vi "Read Lump Data.vi"(8 "Lumps Directory IN":T1[](array[typedef]), 9 "start index (0)":i32, 10 "Lump Name":string, 11 "Input U8":u8[](array[numeric])) -> (0 "Lumps Directory OUT":T1[](array[typedef]), 1 "Lump DATA OUT":u8[](array[numeric]), 2 "Found?":bool, 3 "Output U8":u8[](array[numeric]))   [LabVIEW 2017]
uses:
  Lumps.ctl
panel:
  # "This will check the lump list for the lump name, get the offset and the length on the U8 data file and return the data of the lump"
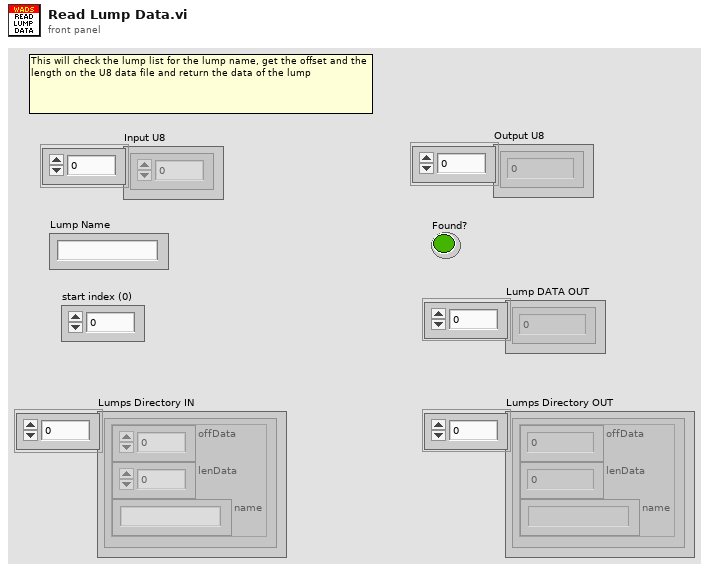
[diagram p1: front panel]
types:
  T1 = typedef "Lumps.ctl" = cluster{"offData":i32, "lenData":i32, "name":string}
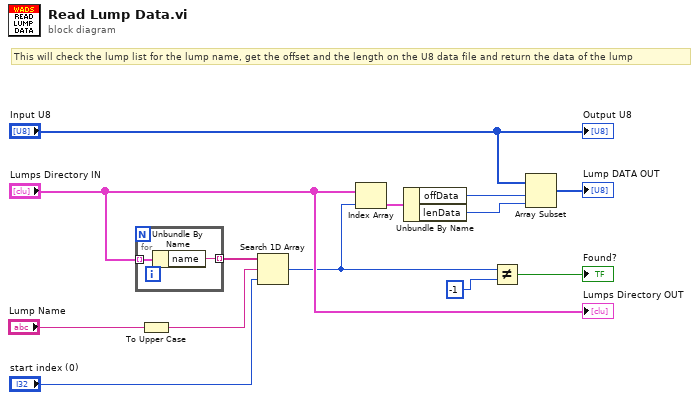
[diagram p0: block diagram]
diagram:
  # "This will check the lump list for the lump name, get the offset and the length on the U8 data file and return the data of the lump"
  n1 = for {
    tunnel: "Lumps Directory IN" -> [w15] mode=indexing
    tunnel: [w14] -> w6 mode=indexing
    n2 = Unbundle By Name(w15) -> ("name"=w14:string)
  }
  n3 = To Upper Case(1:"Lump Name") -> (0:w1:string)
  n4 = Search 1D Array(1D array=w6, element=w1, start index (0)="start index (0)") -> (index of element=w4:i32)
  n5 = Index Array(array="Lumps Directory IN", index=w4) -> (element=w8:T1)
  n6 = Unbundle By Name(w8) -> ("offData"=w10:i32, "lenData"=w11:i32)
  n7 = Not Equal?(x=w4, y=-1) -> (x != y?=→"Found?":bool)
  n8 = Array Subset(array="Input U8", index=w10, length=w11) -> (→"Lump DATA OUT":u8[])
  "Output U8" <- "Input U8"
  "Lumps Directory OUT" <- "Lumps Directory IN"
